vi "svx_Orbit and Timebase Extract (N Ch - 1 Order).vi"(5 "reset? (F)":bool, 6 "segment settings":cluster{"start [rev]":dbl, "end [rev]":dbl}, 8 "error in (no error)":errorcluster, 9 "actual samples/rev in":dbl format="%.2f", 10 "interpolated pulse positions in":dbl[](array[numeric]), 11 "order data in":dbl[][](array[numeric])) -> (0 "error out":errorcluster, 1 "actual samples/rev out":dbl format="%.2f", 2 "interpolated pulse positions out":dbl[](array[numeric]), 3 "order data out":dbl[][](array[numeric]), 4 "end reached":bool)   [LabVIEW 2017]
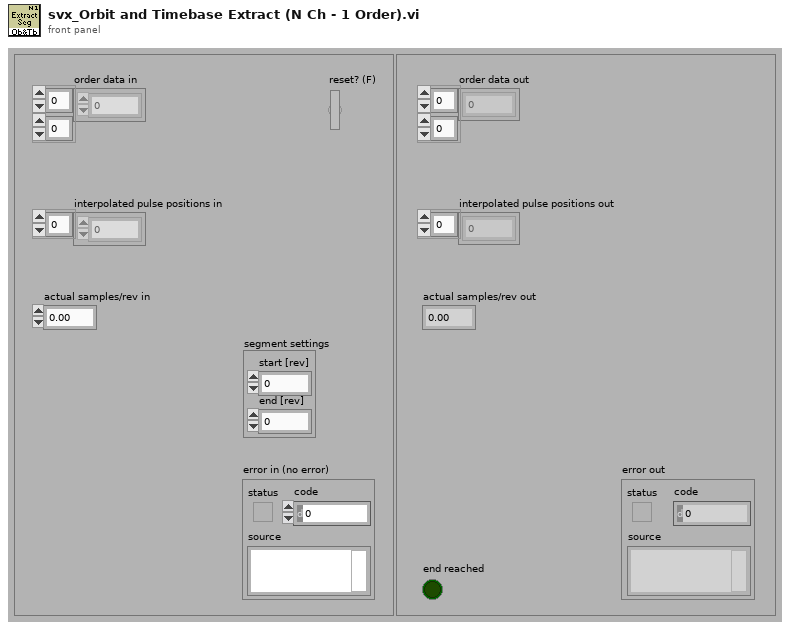
[diagram p1: front panel]
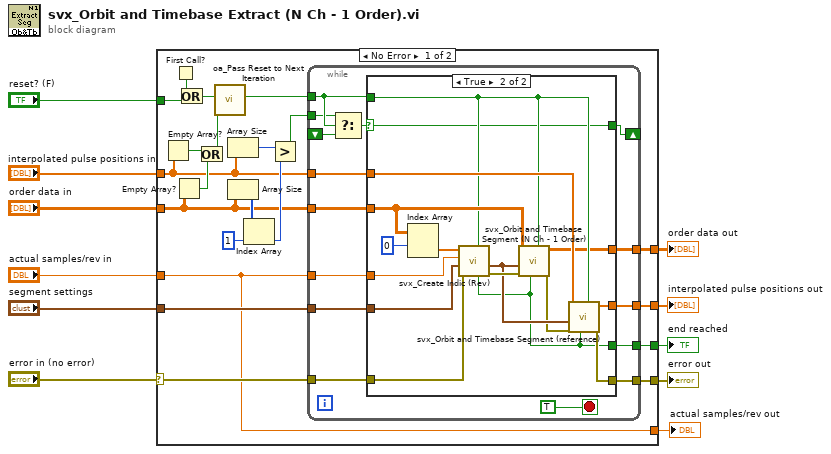
[diagram p0: block diagram]
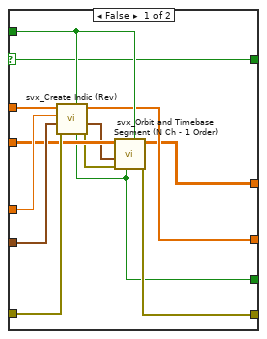
[diagram p2: hidden frame]
diagram:
  n1 = case shown="No Error" "error in (no error)" {
    selector: "error in (no error)" -> [w32 w77]
    tunnel: [w28 w77] -> w10
    tunnel: "reset? (F)" -> [w21 _]
    tunnel: "interpolated pulse positions in" -> [w15 _]
    tunnel: "order data in" -> [w14 _]
    tunnel: "actual samples/rev in" -> [w12 _]
    tunnel: "segment settings" -> [w31 _]
    tunnel: [w30 _] -> w5
    tunnel: [w29 _] -> w4
    tunnel: [w27 _] -> w2
    tunnel: [w12 _] -> w1
    frame No Error {
      n2 = Empty Array?(array=w15) -> (empty?=w24:bool)
      n3 = First Call?() -> (First Call?: T/F=w26:bool)
      n4 = Empty Array?(array=w14) -> (empty?=w23:bool)
      n5 = Or(x=w26, y=w21) -> (x .or. y?=w25:bool)
      n6 = Or(x=w24, y=w23) -> (x .or. y?=w22:bool)
      n7 = call <vilib>:"oa_Pass Reset to Next Iteration.vi"("trigger"=w22, "reset?(F)"=w25) -> ("reset out"=w20:bool)  [unwired: 9 in]
      n8 = Array Size(array=w15) -> (size(s)=w17:i32)
      n9 = Array Size(array=w14) -> (size(s)=w19:i32[])
      n10 = Index Array(array=w19, index=1) -> (element=w16:i32)
      n11 = Greater?(x=w17, y=w16) -> (0:w13:bool)
      n12 = while {
        tunnel: w32 -> [w40]
        shift-right: [w35] -> _
        shift-left: _ -> [w46]
        tunnel: w20 -> [w43]
        tunnel: w15 -> [w39]
        tunnel: w14 -> [w44]
        tunnel: w12 -> [w42]
        tunnel: w31 -> [w41]
        tunnel: [w38] -> w30
        tunnel: [w37] -> w29
        tunnel: [w36] -> w28
        tunnel: [w34] -> w27
        tunnel: w13 -> [w33]
        stop <- TRUE stop-if-true
        n13 = Select(t=w33, s=w43, f=w46) -> (s? t:f=w45:bool)
        n14 = case shown="True" w45 {
          selector: w45 -> [w50 w62]
          tunnel: w44 -> [w56 w70]
          tunnel: w43 -> [w53 w66]
          tunnel: w42 -> [w57 w74]
          tunnel: w41 -> [w58 w73]
          tunnel: w40 -> [w59 w72]
          tunnel: w39 -> [w60 w68]
          tunnel: [w48 w65] -> w38
          tunnel: [w51 w64] -> w37
          tunnel: [w52 w63] -> w36
          tunnel: [w50 w62] -> w35
          tunnel: [w49 w61] -> w34
          frame False {
            n15 = call <vilib>:"svx_Create Indic (Rev).vi"("reset?(F)"=w53, "error in (no error)"=w59, "segment settings"=w58, "actual samples/rev"=w57, "interpolated pulse positions in"=w60) -> ("error out"=w54:errorcluster, "indice"=w55:cluster{"start":i32, "length":i32}, "interpolated pulse positions out"=w51:dbl[], "end reached"=w49:bool)  [unwired: 2 in, 1 out]
            n16 = call <vilib>:"svx_Orbit and Timebase Segment (N Ch - 1 Order).vi"("reset? (F)"=w53, "end reach?"=w49, "error in (no error)"=w54, "indice"=w55, "order data"=w56) -> ("error out"=w52:errorcluster, "order data out"=w48:dbl[][])  [unwired: 5 in]
          }
          frame True {
            n17 = Index Array(array=w70, index (row)=0 ("index (page)")) -> (element=w75:dbl[])  [unwired: 1 in]
            n18 = call <vilib>:"svx_Create Indic (Rev).vi"("reset?(F)"=w66, "error in (no error)"=w72, "segment settings"=w73, "actual samples/rev"=w74, "interpolated pulse positions in"=w75) -> ("error out"=w71:errorcluster, "indice"=w69:cluster{"start":i32, "length":i32}, "end reached"=w61:bool)  [unwired: 2 in, 2 out]
            n19 = call <vilib>:"svx_Orbit and Timebase Segment (N Ch - 1 Order).vi"("reset? (F)"=w66, "end reach?"=w61, "error in (no error)"=w71, "indice"=w69, "order data"=w70) -> ("error out"=w67:errorcluster, "order data out"=w65:dbl[][])  [unwired: 5 in]
            n20 = call <vilib>:"svx_Orbit and Timebase Segment (reference).vi"("reset? (F)"=w66, "end reach?"=w61, "error in (no error)"=w67, "indice"=w69, "order data"=w68) -> ("error out"=w63:errorcluster, "order data out"=w64:dbl[])  [unwired: 5 in]
          }
        }
      }
    }
    frame Error {
    }
  }
  "error out" <- w10
  "interpolated pulse positions out" <- w4
  "order data out" <- w5
  "actual samples/rev out" <- w1
  "end reached" <- w2
